vi "Diag_SeqInfo.vi"(0 "GEA2 Reference In":refnum<k24>, 5 "GEA Inputs":T3={"Source"=228, "Destination"=0} {"Destination" format="%.0x"; "Source" format="%.0x"}, 7 "Seq Status Location":u16 format="%.0x", 9 "Seq Entry Count":u16, 11 "Error In":errorcluster) -> (4 "GEA2 Reference Out":refnum<k24>, 6 "Fault Seq Status":T2, 8 "Fault Sequence Entries":T1[](array[typedef]), 15 "Error Out":errorcluster)   [LabVIEW 2023]
uses:
  D:/Common/LabVIEW GEA2 Toolkit/source/GEA3 DLL Source/GeaCommunication.dll
  LabVIEW GEA2 Toolkit/source/GEA3 DLL Source/GeaCommunication.dll
  LabVIEW GEA2 Toolkit/GEA3/type defs/Source_Destination.ctl
  Type Defs/Diag_FaultTableStatus.ctl
  Type Defs/Diag_FaultSeqEntry.ctl
  LabVIEW GEA2 Toolkit/GEA3/type defs/ERD Read Data In.ctl
  LabVIEW GEA2 Toolkit/GEA3/library/GEA2_Toolkit.lvlib
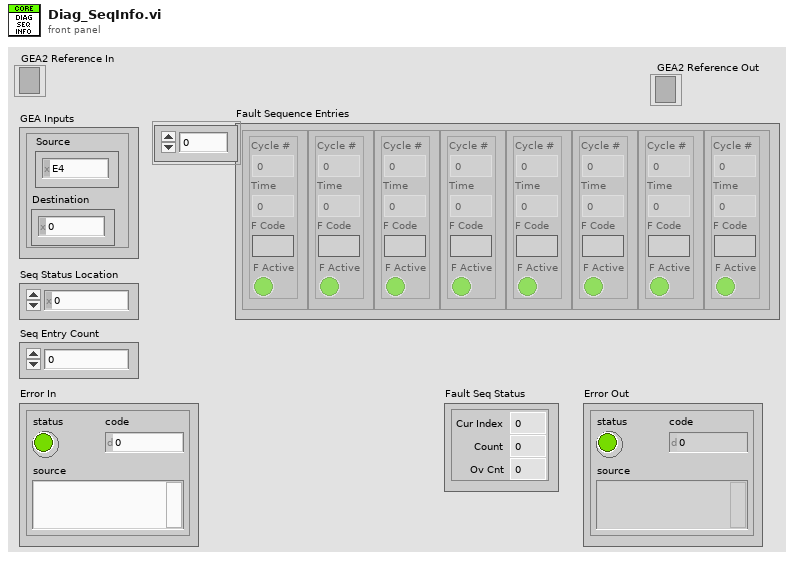
[diagram p1: front panel]
types:
  T1 = typedef "Diag_FaultSeqEntry.ctl" = cluster{"Cycle #":u32, "Time":u32, "F Code":string, "F Active":bool}
  T2 = typedef "Diag_FaultTableStatus.ctl" = cluster{"Cur Index":u16, "Count":u16, "Ov Cnt":u16}
  T3 = typedef "Source_Destination.ctl" = cluster{"Source":u8, "Destination":u8}
  T4 = typedef "ERD Read Data In.ctl" = cluster{"ERD Number":u16, "Data Type":enum16{"string", "boolean", "uint8_t", "uint16_t", "uint32_t", "uint64_t", "int8_t", "int16_t", "int32_t", "int64_t"}}
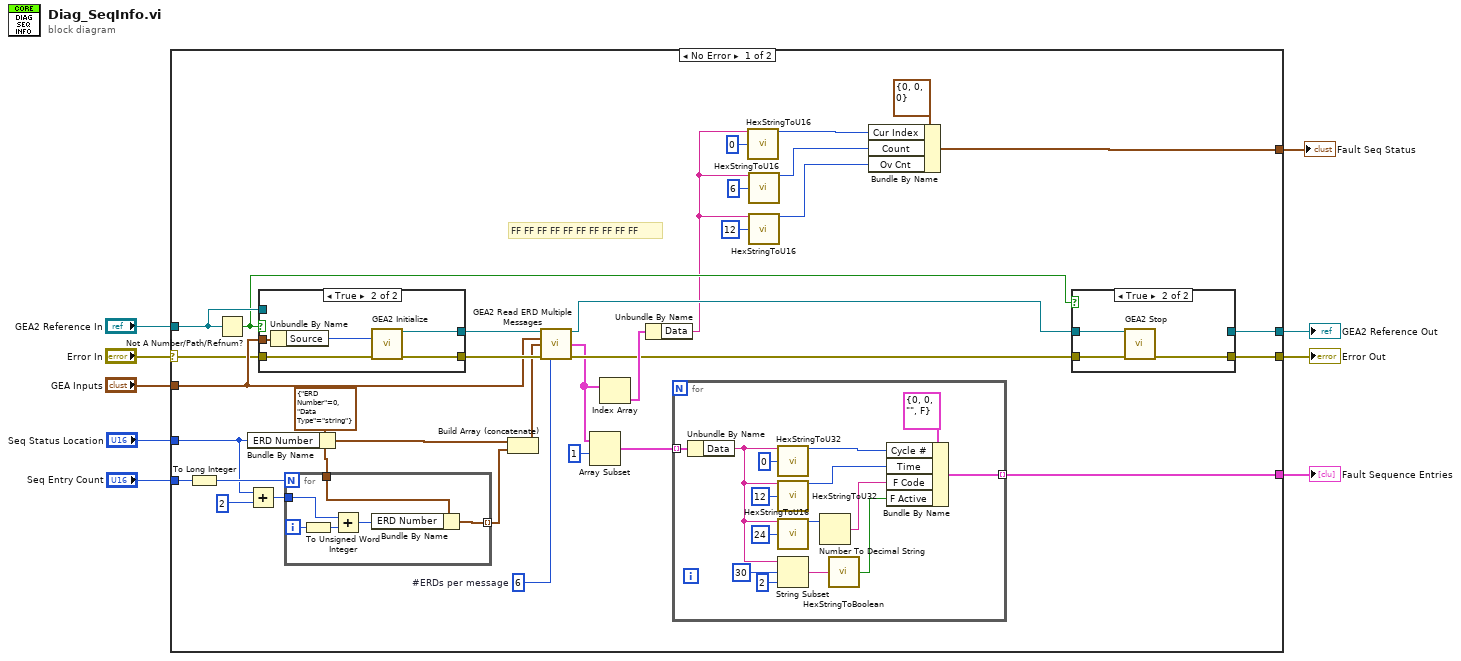
[diagram p0: block diagram]
diagram:
  n1 = case shown="No Error" "Error In" {
    selector: "Error In" -> [w35 w78]
    tunnel: [w34 w78] -> w9
    tunnel: "GEA2 Reference In" -> [w43 w77]
    tunnel: "GEA Inputs" -> [w39 _]
    tunnel: [w36 w77] -> w6
    tunnel: "Seq Status Location" -> [w12 _]
    tunnel: "Seq Entry Count" -> [w14 _]
    tunnel: [w16 _] -> w2
    tunnel: [w10 _] -> w1
    frame No Error {
      w28 = 6  # #ERDs per message
      w30 = T4 {"ERD Number"=0, "Data Type"=enum."string"} ("ERD Read Data In")
      # "FF FF FF FF FF FF FF FF FF FF"
      n2 = To Long Integer(number=w14) -> (32bit integer=w13:i32)
      n3 = Not A Number/Path/Refnum?(number/path/refnum=w43) -> (NaN/Path/Refnum?=w37:bool)
      n4 = Bundle By Name(cluster=w30, "ERD Number"=w12) -> (w29:T4)
      n5 = Add(x=w12, y=u16 2 ("x")) -> (x+y=w31:u16)
      n6 = case shown="True" w37 {
        tunnel: w35 -> [w70 w76]
        tunnel: w39 -> [_ w75]
        tunnel: [w70 w74] -> w42
        tunnel: [w71 w73] -> w41
        tunnel: w43 -> [w71 _]
        frame False {
        }
        frame True {
          n7 = Unbundle By Name(w75) -> ("Source"=w72:u8)
          n8 = call "GEA2 Initialize.vi"("Source Address"=w72, "error in"=w76) -> ("GEA2 Reference Out"=w73:refnum<k24>, "error out"=w74:errorcluster)  [unwired: 10 in, 2 out]
        }
      }
      n9 = for {
        N: w13 -> [_]
        tunnel: w31 -> [w62]
        tunnel: w30 -> [w64]
        tunnel: [w63] -> w11 mode=indexing
        i -> [w59]
        n10 = To Unsigned Word Integer(number=w59) -> (unsigned 16bit integer=w60:u16)
        n11 = Add(x=w62, y=w60) -> (x+y=w61:u16)
        n12 = Bundle By Name(cluster=w64, "ERD Number"=w61) -> (w63:T4)
      }
      n13 = Build Array (concatenate)(w29, w11) -> (w27:T4[])
      n14 = call "GEA2 Read ERD Multiple Messages.vi"("GEA2 Reference In"=w41, "GEA Inputs"=w39, "Read ERD List"=w27, "Error In"=w42, "#ERDs per message"=w28) -> ("GEA2 Reference Out"=w38:refnum<k24>, "ERD Data Out"=w26:cluster{"ERD Number":u16, "Data":string}[], "Error Out"=w33:errorcluster)  [unwired: 7 in, 1 out]
      n15 = Array Subset(array=w26, index=1) -> (w15:cluster{"ERD Number":u16, "Data":string}[])  [unwired: 1 in]
      n16 = Index Array(array=w26) -> (element=w40:cluster{"ERD Number":u16, "Data":string})  [unwired: 1 in]
      n17 = Unbundle By Name(w40) -> ("Data"=w20:string)
      n18 = for {
        tunnel: w15 -> [w58] mode=indexing
        tunnel: [w44] -> w10 mode=indexing
        n19 = Unbundle By Name(w58) -> ("Data"=w55:string)
        n20 = call "HexStringToU32.vi"("Input String"=w55, "Starting Offset"=0) -> ("Number Out"=w48:u32)  [unwired: 13 in]
        n21 = call "HexStringToU32.vi"("Input String"=w55, "Starting Offset"=12) -> ("Number Out"=w47:u32)  [unwired: 13 in]
        n22 = call "HexStringToU16.vi"("Input String"=w55, "Starting Offset"=24) -> ("Number Out"=w51:u16)  [unwired: 13 in]
        n23 = String Subset(string=w55, offset (0)=30, length (rest)=2 ("length (rest)")) -> (substring=w54:string)
        n24 = Number To Decimal String(number=w51) -> (decimal integer string=w46:string)  [unwired: 1 in]
        n25 = call "HexStringToBoolean.vi"("Hex String"=w54) -> ("Boolean"=w45:bool)
        n26 = Bundle By Name(cluster=T1 {"Cycle #"=0, "Time"=0, "F Code"="", "F Active"=FALSE} ("Fault Entry 1"), "Cycle #"=w48, "Time"=w47, "F Code"=w46, "F Active"=w45) -> (w44:T1)
      }
      n27 = call "HexStringToU16.vi"("Input String"=w20, "Starting Offset"=0) -> ("Number Out"=w19:u16)  [unwired: 13 in]
      n28 = call "HexStringToU16.vi"("Input String"=w20, "Starting Offset"=6) -> ("Number Out"=w18:u16)  [unwired: 13 in]
      n29 = call "HexStringToU16.vi"("Input String"=w20, "Starting Offset"=12) -> ("Number Out"=w17:u16)  [unwired: 13 in]
      n30 = Bundle By Name(cluster=T2 {"Cur Index"=0, "Count"=0, "Ov Cnt"=0} ("Fault Table Status"), "Cur Index"=w19, "Count"=w18, "Ov Cnt"=w17) -> (w16:T2)
      n31 = case shown="True" w37 {
        tunnel: w33 -> [w65 w69]
        tunnel: [w65 w68] -> w34
        tunnel: [w66 _] -> w36
        tunnel: w38 -> [w66 w67]
        frame False {
        }
        frame True {
          n32 = call "GEA2 Stop.vi"("GEA2 Reference In"=w67, "Error In"=w69) -> ("Error Out"=w68:errorcluster)  [unwired: 13 in]
        }
      }
    }
    frame Error {
    }
  }
  "Error Out" <- w9
  "GEA2 Reference Out" <- w6
  "Fault Seq Status" <- w2
  "Fault Sequence Entries" <- w1
